vi "Get Terminal Name.vi"(8 "error in":errorcluster, 11 "remote terminal in":T1 format="%.0x") -> (0 "error out":errorcluster, 2 "terminal name":string, 3 "remote terminal out":T1 format="%.0x")   [LabVIEW 2020, in "AIM MIL-STD-1553 Scripting.lvlib"]
doc: "Gets the terminal name of the input <b>remote terminal in</b>."
uses:
  AIM MIL-STD-1553 Scripting.lvlib
  <vilib>/NI VeriStand/Custom Device API/Custom Device Item Ref.ctl
  <vilib>/NI VeriStand/Custom Device API/Custom Device API.lvlib
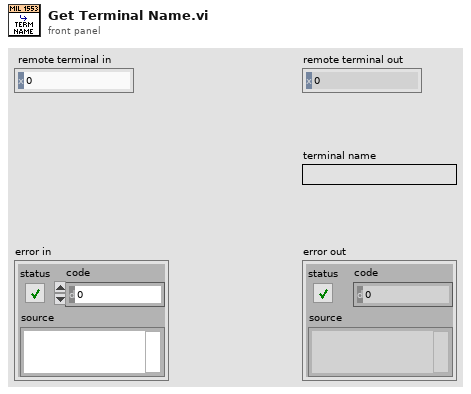
[diagram p1: front panel]
types:
  T1 = typedef "Custom Device API.lvlib/Custom Device Item Ref.ctl" = u64
  T2 = typedef "Custom Device API.lvlib/Custom Device Item Info.ctl" = cluster{"Name":string, "Is Channel":bool, "GUID":string, "Is Waveform":bool}
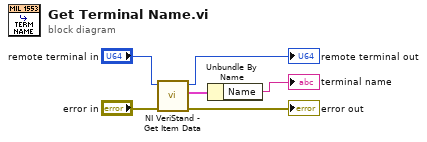
[diagram p0: block diagram]
diagram:
  n1 = call <vilib>:"NI VeriStand - Get Item Data.vi"("error in (no error)"="error in", "Item Ref in"="remote terminal in") -> ("error out"=→"error out":errorcluster, "Item Info"=w6:T2, "Item Ref out"=→"remote terminal out":T1)  [unwired: 6 in, 1 out]
  n2 = Unbundle By Name(w6) -> ("Name"=→"terminal name":string)
